vi "Global MT valvola motorizz.vi"() -> ()   [LabVIEW 2016]
panel:
  out "Magnetot valvola motor":bool
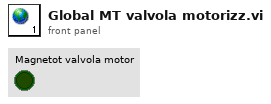
[diagram p1: front panel]
diagram:
